vi "logistic_MODCA.vi"(3 "output control":T1, 4 "data":variant, 5 "X":dbl[](array[numeric]), 6 "a":dbl[](array[numeric])) -> (0 "error out":errorcluster, 1 "f'(X,a)":dbl[][](array[numeric]), 2 "f(X,a)":dbl[](array[numeric]))   [LabVIEW 2014]
doc: "This template is the starting point for creating a model function to be passed to the Nonlinear Curve Fit.vi."
uses:
  <vilib>/gmath/NumericalOptimization/LM_output select.ctl
  <vilib>/gmath/NI_Gmath.lvlib
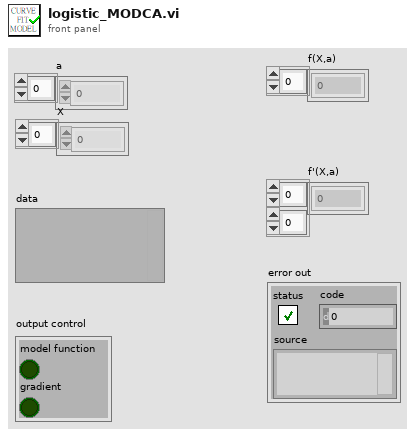
[diagram p1: front panel]
types:
  T1 = typedef "NI_Gmath.lvlib/LM_output select.ctl" = cluster{"model function":bool, "gradient":bool}
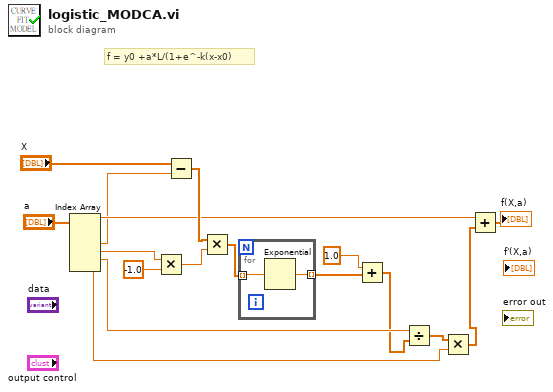
[diagram p0: block diagram]
diagram:
  # "f = y0 +a*L/(1+e^-k(x-x0)"
  n1 = Index Array(array="a") -> (element #1=w13:dbl, element #2=w12:dbl, element #3=w10:dbl, element #4=w6:dbl, element #5=w3:dbl)  [unwired: 5 in]
  n2 = Multiply(x=w10, y=-1.0) -> (x*y=w9:dbl)
  n3 = Subtract(x="X", y=w12) -> (x-y=w15:dbl[])
  n4 = Multiply(x=w15, y=w9) -> (x*y=w14:dbl[])
  n5 = for {
    tunnel: w14 -> [w19] mode=indexing
    tunnel: [w18] -> w8 mode=indexing
    n6 = Exponential(1:w19) -> (0:w18:dbl)
  }
  n7 = Add(x=1.0 ("y"), y=w8) -> (x+y=w5:dbl[])
  n8 = Divide(x=w6, y=w5) -> (x/y=w4:dbl[])
  n9 = Multiply(x=w4, y=w3) -> (x*y=w2:dbl[])
  n10 = Add(x=w13, y=w2) -> (x+y=→"f(X,a)":dbl[])
